vi "Configure osciloscopio FULL.vi"(0 "Visa MDO3104":refnum<visa-resource-name>="Osciloscopio_Tek_MDO3104", 5 "Valor VGA":u8=115, 7 "V reference":dbl=1.0096, 9 "Tolerance":dbl=10.0 format="%#_g%%", 11 "error out":errorcluster, 12 "Esperar a completar estadisticas":bool, 13 "Configurar Osciloscopio":bool=TRUE) -> (4 "VISA resource name out 2":refnum<visa-resource-name>="Osciloscopio_Tek_MDO3104", 6 "Array":dbl[](array[numeric])=[0.4730278, 0.4040874, 0.8764885, 3.0701e-09], 8 "Ch1+Ch2":dbl=0.8771152, 10 "Math (CH1-CH2)":dbl=0.8764885, 15 "error out 2":errorcluster)   [LabVIEW 2009]
doc: "Atencion!!!!\nEl osciloscopio algunas veces no consigue medir correctamente la funcion matematica dando valores de tension por debajo del que muestra la pantalla y un ancho de pulso de infinito.\nPor ello hay dos salidas Ch1+Ch2 que seria la suma de las medias de las amplitudes de ambos canales o bien Math (ch1-ch2) que seria la media de las resta punto a punto de los dos canales.\nGustavo piensa que es mejor MATH yo creo que es mejor la otra ya veremos como la cableo."
uses:
  <instrlib>/Tektronix DPO MSO 2000 4000 Series/Tektronix DPO MSO 2000 4000 Series.lvlib
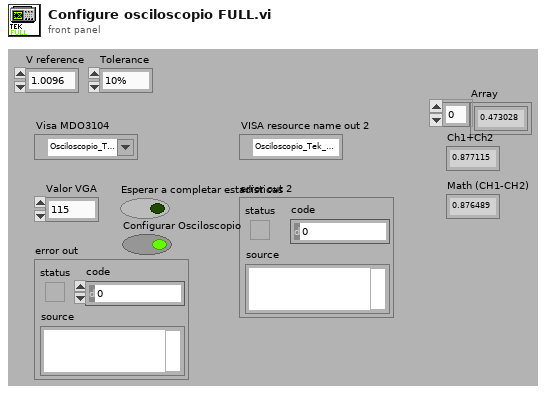
[diagram p1: front panel]
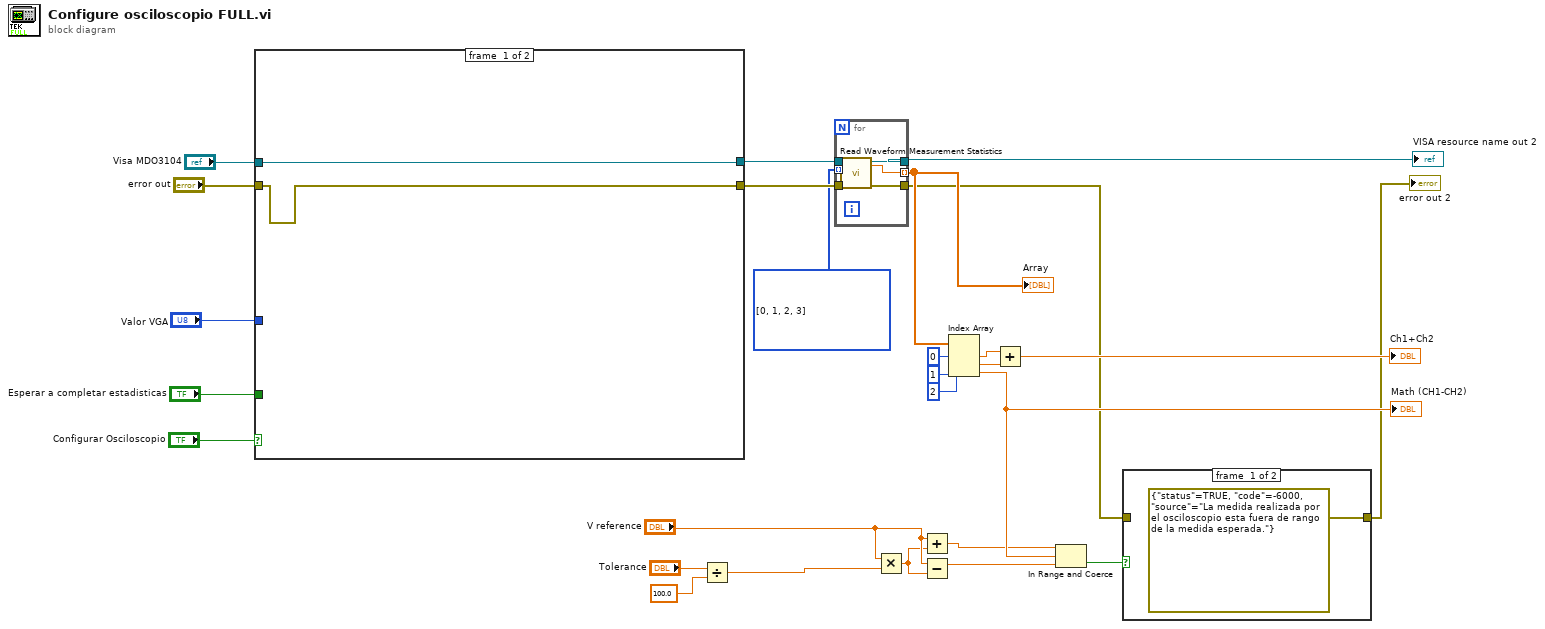
[diagram p0: block diagram]
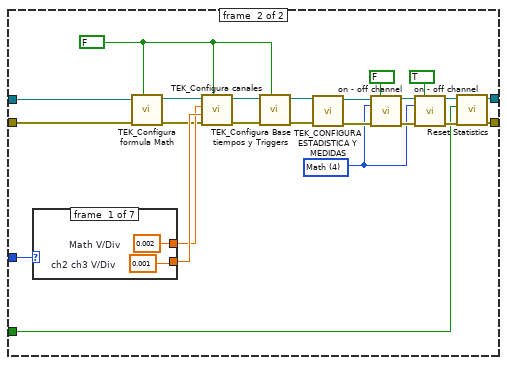
[diagram p2: hidden frame]
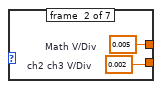
[diagram p3: hidden frame]
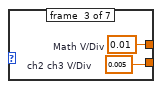
[diagram p4: hidden frame]
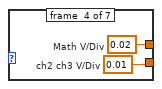
[diagram p5: hidden frame]
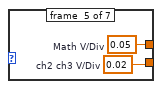
[diagram p6: hidden frame]
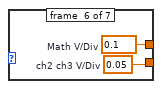
[diagram p7: hidden frame]
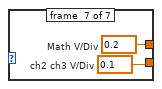
[diagram p8: hidden frame]
diagram:
  w22 = i32[] [0, 1, 2, 3] items=["Measurement 1", "Measurement 2", "Measurement 3", "Measurement 4"]
  n1 = case shown="True" "Configurar Osciloscopio" {
    tunnel: "Valor VGA" -> [_ w52]
    tunnel: "error out" -> [w28 w49]
    tunnel: "Visa MDO3104" -> [w29 w48]
    tunnel: [w28 w41] -> w24
    tunnel: [w29 w40] -> w23
    tunnel: "Esperar a completar estadisticas" -> [_ w30]
    frame #0 {
    }
    frame #1 {
      w31 = u16 4 items=["Channel 1", "Channel 2", "Channel 3", "Channel 4", "Math", "Reference 1", "Reference 2", "Reference 3", "Reference 4", "Bus 1", "Bus 2"] ("Channel (0: Channel 1)")
      w53 = FALSE ("Debug")
      n2 = case shown="3..6" w52 {
        tunnel: [w55 w57 w59 w61 w63 w65 w67] -> w50
        tunnel: [w54 w56 w58 w60 w62 w64 w66] -> w51
        frame #0 {
          w54 = 0.001  # ch2 ch3 V/Div
          w55 = 0.002  # Math V/Div
        }
        frame #1 {
          w56 = 0.002  # ch2 ch3 V/Div
          w57 = 0.005  # Math V/Div
        }
        frame #2 {
          w58 = 0.005  # ch2 ch3 V/Div
          w59 = 0.01  # Math V/Div
        }
        frame #3 {
          w60 = 0.01  # ch2 ch3 V/Div
          w61 = 0.02  # Math V/Div
        }
        frame #4 {
          w62 = 0.02  # ch2 ch3 V/Div
          w63 = 0.05  # Math V/Div
        }
        frame #5 {
          w64 = 0.05  # ch2 ch3 V/Div
          w65 = 0.1  # Math V/Div
        }
        frame #6 {
          w66 = 0.1  # ch2 ch3 V/Div
          w67 = 0.2  # Math V/Div
        }
      }
      n3 = call "TEK_Configura formula Math.vi"("Debug"=w53, "error out"=w49, "VISA resource name out 2"=w48) -> ("error out 2"=w44:errorcluster, "VISA resource name out"=w45:refnum<visa-resource-name>)  [unwired: 7 in]
      n4 = call "TEK_Configura canales.vi"("Debug"=w53, "error out 2"=w44, "ch2 ch3 V/Div"=w51, "Math V/Div"=w50, "VISA resource name out"=w45) -> ("error out"=w47:errorcluster, "VISA resource name out 2"=w46:refnum<visa-resource-name>)  [unwired: 5 in]
      n5 = call "TEK_Configura Base tiempos y Triggers.vi"("Debug"=w53, "error out 2"=w47, "VISA resource name out 2"=w46) -> ("error out"=w42:errorcluster, "VISA resource name out"=w43:refnum<visa-resource-name>)  [unwired: 7 in]
      n6 = call "TEK_CONFIGURA ESTADISTICA Y MEDIDAS.vi"("error out"=w42, "VISA resource name out"=w43) -> ("error out 2"=w32:errorcluster, "VISA resource name out 2"=w33:refnum<visa-resource-name>)  [unwired: 8 in]
      n7 = call "on - off channel.vi"("VISA resource name"=w33, "Enable Channel (T: Enable)"=FALSE, "Channel (0: Channel 1)"=w31, "error in (no error)"=w32) -> ("VISA resource name out"=w39:refnum<visa-resource-name>, "error out"=w38:errorcluster)  [unwired: 10 in]
      n8 = call "on - off channel.vi"("VISA resource name"=w39, "Enable Channel (T: Enable)"=TRUE, "Channel (0: Channel 1)"=w31, "error in (no error)"=w38) -> ("VISA resource name out"=w36:refnum<visa-resource-name>, "error out"=w37:errorcluster)  [unwired: 10 in]
      n9 = call "Reset Statistics.vi"("error in (no error)"=w37, "Wait medida"=w30, "VISA resource name"=w36) -> ("error out"=w41:errorcluster, "VISA resource name out"=w40:refnum<visa-resource-name>)  [unwired: 7 in]
    }
  }
  n10 = Divide(x="Tolerance", y=100.0) -> (x/y=w6:dbl)
  n11 = for {
    tunnel: [w73] -> w4
    tunnel: [w72] -> w21
    tunnel: [w71] -> w20 mode=indexing
    tunnel: w24 -> [w70]
    tunnel: w23 -> [w69]
    tunnel: w22 -> [w68] mode=indexing
    n12 = call <instrlib>:"Read Waveform Measurement Statistics.vi"("error in (no error)"=w70, "Measurement Number (0: Measurement 1)"=w68, "VISA resource name"=w69) -> ("error out"=w73:errorcluster, "VISA resource name out"=w72:refnum<visa-resource-name>, "Mean Value"=w71:dbl)  [unwired: 3 in, 3 out]
  }
  "VISA resource name out 2" <- w21
  "Array" <- w20
  n13 = Multiply(x="V reference", y=w6) -> (x*y=w11:dbl)
  n14 = Add(x="V reference", y=w11) -> (x+y=w10:dbl)
  n15 = Subtract(x="V reference", y=w11) -> (x-y=w9:dbl)
  n16 = Index Array(array=w20, index #1=0 ("index"), index #2=1 ("index"), index #3=2 ("index")) -> (element #1=w16:dbl, element #2=w15:dbl, element #3=w13:dbl)
  "Math (CH1-CH2)" <- w13
  n17 = Add(x=w16, y=w15) -> (x+y=→"Ch1+Ch2":dbl)
  n18 = In Range and Coerce(upper limit=w10, x=w13, lower limit=w9) -> (In Range?=w5:bool)  [unwired: 1 out]
  n19 = case shown="False" w5 {
    tunnel: w4 -> [_ w75]
    tunnel: [errorcluster {"status"=TRUE, "code"=-6000, "source"="La medida realizada por el osciloscopio esta fuera de rango de la medida esperada."} ("error out") w75] -> w3
    frame #0 {
    }
    frame #1 {
    }
  }
  "error out 2" <- w3
